vi "MSG Stop.vi"(8 "error in":errorcluster) -> (0 "error out":errorcluster)   [LabVIEW 2020, in "GUI.lvlib"]
uses:
  GUI.lvlib
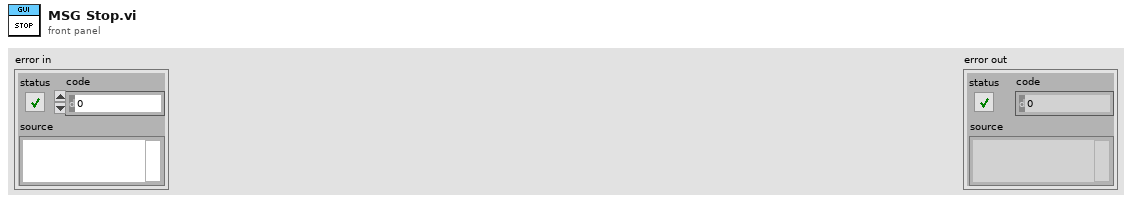
[diagram p1: front panel]
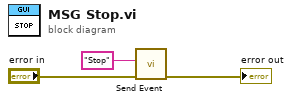
[diagram p0: block diagram]
diagram:
  n1 = call "Send Event.vi"("error in"="error in", "Command"="Stop") -> ("error out"=→"error out":errorcluster)  [unwired: 9 in]
